vi "Personlist.vi"() -> ()   [LabVIEW 2020]
uses:
  PL_Global.vi
panel:
  in  "stop":bool
  in  "PERSON LIST":T1={"NAMES"=["USERNAME1", "USERNAME2", "USERNAME3", "USERNAME4", "USERNAME5", "USERNAME6", "USERNAME7", "USERNAME8", "USERNAME9", "USERNAME10", "USERNAME11", "USERNAME12", "USERNAME13", "USERNAME14", "USERNAME15"], "ID"=[20001.0, 20002.0, 20003.0, 20004.0, 20005.0, 20006.0, 20007.0, 20008.0, 20009.0, 20010.0, 20011.0, 20012.0, 20013.0, 20014.0, 20015.0], "PASSWORD"=["PASSWORD1", "PASSWORD2", "PASSWORD3", "PASSWORD4", "PASSWORD5", "PASSWORD6", "PASSWORD7", "PASSWORD8", "PASSWORD9", "PASSWORD10", "PASSWORD11", "PASSWORD12", "PASSWORD13", "PASSWORD14", "PASSWORD15"]}
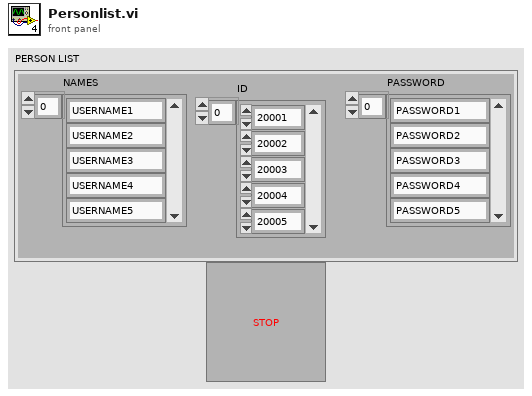
[diagram p1: front panel]
types:
  T1 = cluster{"NAMES":string[], "ID":dbl[], "PASSWORD":string[]}
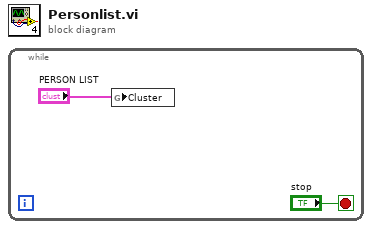
[diagram p0: block diagram]
diagram:
  n1 = while {
    stop <- "stop" stop-if-true
    n2 = global write "PL_Global.vi" "Cluster"("PERSON LIST") -> ()
  }
